vi "Admin.vi"(2 "Admin File Directory":string="C:\\Setup Files\\", 3 "MFC Error":u32) -> ()   [LabVIEW 2014]
uses:
  Program Files (x86)/National Instruments/LabVIEW 2014/examples/CompactRIO/Shared/cRIO Convert Thermocouple Readings.llb/Thermocouple Type.ctl
  <vilib>/Utility/file.llb/Read From Spreadsheet File (DBL).vi
  <vilib>/Utility/file.llb/Read From Spreadsheet File (string).vi
  <vilib>/Utility/file.llb/Write To Spreadsheet File (DBL).vi
  <vilib>/Utility/file.llb/Write To Spreadsheet File (string).vi
  <vilib>/Utility/file.llb/Write To Spreadsheet File (I64).vi
panel:
  in  "MKS 2":bool
  in  "IP Address MKS 2030 2":string
  in  "Mexa One":bool
  in  "IP Address Mexa One":string
  in  "Rapidox":bool
  in  "Mexa 584 - 2":bool
  in  "Mexa 584":bool
  out "PID Array":dbl[](array[numeric])
  out "Output array":u32[](array[numeric])
  out "IP array":string[](array[string])
  out "Boolean":bool
  in  "OK Button":bool
  in  "Tab Control":T1(tab)
  in  "Fast Warmup":bool
  in  "Omega":bool
  in  "Drive Cycle":bool
  in  "Ageing":bool
  in  "OSC Test":bool
  in  "AFR Sweep":bool
  in  "NO Light Off":bool
  in  "HC Light Off":bool
  in  "CO Light Off":bool
  in  "Heat Load Control":bool
  in  "Array Injection":bool
  in  "D SO2":dbl min=0.0 max=100.0
  in  "I SO2":dbl min=0.0 max=100.0
  in  "P SO2":dbl min=0.0 max=100.0
  in  "D NO":dbl min=0.0 max=100.0
  in  "I NO":dbl min=0.0 max=100.0
  in  "P NO":dbl min=0.0 max=100.0
  in  "D Fan":dbl min=0.0 max=100.0
  in  "I Fan":dbl min=0.0 max=100.0
  in  "P Fan":dbl min=0.0 max=100.0
  in  "D Furnace":dbl min=0.0 max=100.0
  in  "I Furnace":dbl min=0.0 max=100.0
  in  "P Furnace":dbl min=0.0 max=100.0
  in  "SO2 Loop":bool
  in  "CO2 Loop":bool
  in  "NO Loop":bool
  in  "Air Loop":bool
  in  "CO Loop":bool
  in  "HC Loop":bool
  in  "N2 Loop":bool
  in  "Air B Loop":bool
  in  "Air 2 Loop":bool
  in  "HC 2 Loop":bool
  in  "HC B Loop":bool
  out "CO -Al":bool
  out "HC - AL":bool
  out "AIR-Al":bool
  out "NO - AL":bool
  out "N2 - AL":bool
  out "SO2 AL":bool
  out "CO2 -Al":bool
  in  "HC-B Size":i32 min=0 max=100
  in  "Air-B Size":i32 min=0 max=5000
  in  "N2 Size":i32 min=0 max=1000
  in  "NO Size":i32 min=0 max=100
  in  "Air Size":i32 min=0 max=5000
  in  "HC Size":i32 min=0 max=100
  in  "CO Size":i32 min=0 max=100
  in  "N2-2 Size":i32 min=0 max=1000
  in  "Air-2 Size":i32 min=0 max=1000
  in  "HC-2 Size":i32 min=0 max=5000
  in  "O2 Size":i32 min=0 max=1000
  out "HC 2 - AL":bool
  out "Air 2 - AL":bool
  out "HC B -Al":bool
  out "Air B - AL":bool
  in  "SO2 F":bool
  in  "CO2 F":bool
  in  "NO F":bool
  in  "Air F":bool
  in  "CO F":bool
  in  "HC F":bool
  in  "N2 F":bool
  in  "Air B F":bool
  in  "Air 2 F":bool
  in  "HC 2 F":bool
  in  "HC B F":bool
  in  "HC-B":bool
  in  "N2":bool
  in  "NO":bool
  in  "Air":bool
  in  "CO":bool
  in  "HC":bool
  in  "Air-B":bool
  in  "Air-2":bool
  in  "HC-2":bool
  in  "O2":bool
  in  "N2-2":bool
  in  "Tank Thermocouple Limit":i32=300 min=0 max=1372
  in  "Heat Exch D":i32=1 min=0 max=32
  in  "Heat Exch C":i32=1 min=0 max=32
  in  "Heat Exch B":i32=1 min=0 max=32
  in  "Heat Exch A":i32=1 min=0 max=32
  in  "Vane Wheel":i32=1 min=0 max=32
  in  "Venturi":i32=1 min=0 max=32
  in  "Mopup Thermocouple":i32 min=0 max=32
  in  "Tank Thermocouple":i32 min=0 max=32
  in  "Process Thermocouple":i32=1 min=0 max=32
  in  "Process Thermocouple Limit":i32 min=0 max=1372
  in  "Bearing Temperature Limit":i32 min=0 max=200
  in  "Machine Temperature Limit":i32 min=0 max=1375
  in  "Bearing 1 TC":i32 min=0 max=32
  in  "Bearing 2 TC":i32 min=0 max=32
  in  "TC_Type_Array":T2[](array[typedef])=[3, 3, 3, 3, 3, 3, 3, 3, 3, 3, 3, 3, 3, 3, 3, 3] items=["B", "E", "J", "K", "R", "S", "T", "N"]
  in  "CO2 PS":bool
  in  "N2 PS":bool
  in  "CO PS":bool
  in  "HC PS":bool
  in  "Air-B/SO2 PS":bool
  in  "NO PS":bool
  in  "Air PS":bool
  in  "NO2 GLD":bool
  in  "SO2 GLD":bool
  in  "HC GLD":bool
  in  "CO GLD":bool
  in  "Inverter Err":bool
  in  "eStop":bool
  in  "ETAS":bool
  in  "IP Address ETAS":string
  in  "Port MKS":string
  in  "Port Mexa 7000-3":string
  in  "Port Mexa 7000-2":string
  in  "Port Mexa 7000-1":string
  in  "Mexa 7000-3":bool
  in  "IP Address Mexa 7000-3":string
  in  "Mexa 7000-2":bool
  in  "IP Address Mexa 7000-2":string
  in  "Mexa 7170":bool
  in  "MKS":bool
  in  "IP Address MKS 2030":string
  in  "IP Address Mexa 7000-1":string
  in  "Pressure Leak Test":i32 min=0 max=100
  in  "Delivery":i32 min=0 max=100
  in  "Air Bal":bool
  in  "N2 Leak":bool
  in  "Duration Leak Test":i32 min=0 max=100
  # "System Settings"
  # "Omicron"
  # "PID Settings"
  # "NO"
  # "Furnace"
  # "Fan"
  # "SO2"
  # "MFC Settings"
  # "Connected ?"
  # "Alarm"
  # "Size"
  # "Factors"
  # "Fast Loop"
  # "TC Settings"
  # "°C"
  # "°C"
  # "°C"
  # "°C"
  # "Flow Thermocouples"
  # "Heat Exchanger Thermocouples"
  # "TC Type"
  # "TC 01"
  # "TC 02"
  # "TC 03"
  # "When Selecting TC type PLEASE ensure the TC is wired with the correct wire back to the NI 9213 Module\n\nType: K Green (Default)\n          S Orange (Usually Furnace)\n          N Pink"
  # "TC 04"
  # "TC 05"
  # "TC 06"
  # "TC 07"
  # "TC 08"
  # "TC 09"
  # "TC 10"
  # "TC 11"
  # "TC 12"
  # "TC 13"
  # "TC 14"
  # "TC 15"
  # "TC 16"
  # "Alarm Settings"
  # "Analyser Settings"
  # "IP Address"
  # "Port Number"
  # "Leak Test Settings"
  # "KPa"
  # "s"
  # "l/min"
  # "Gas to be Used"
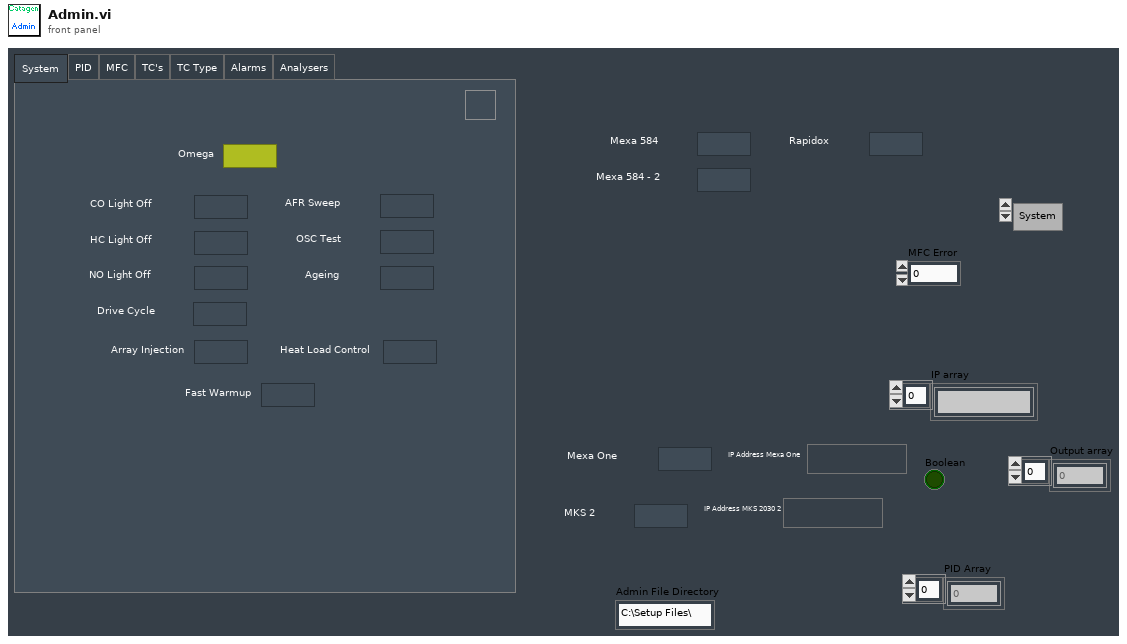
[diagram p1: front panel]
types:
  T1 = enum32{"System ", "Furnace", "MFC", "TC's", "TC Type", "Alarms", "Analysers", "Leak Test"}
  T2 = typedef "Thermocouple Type.ctl" = u16
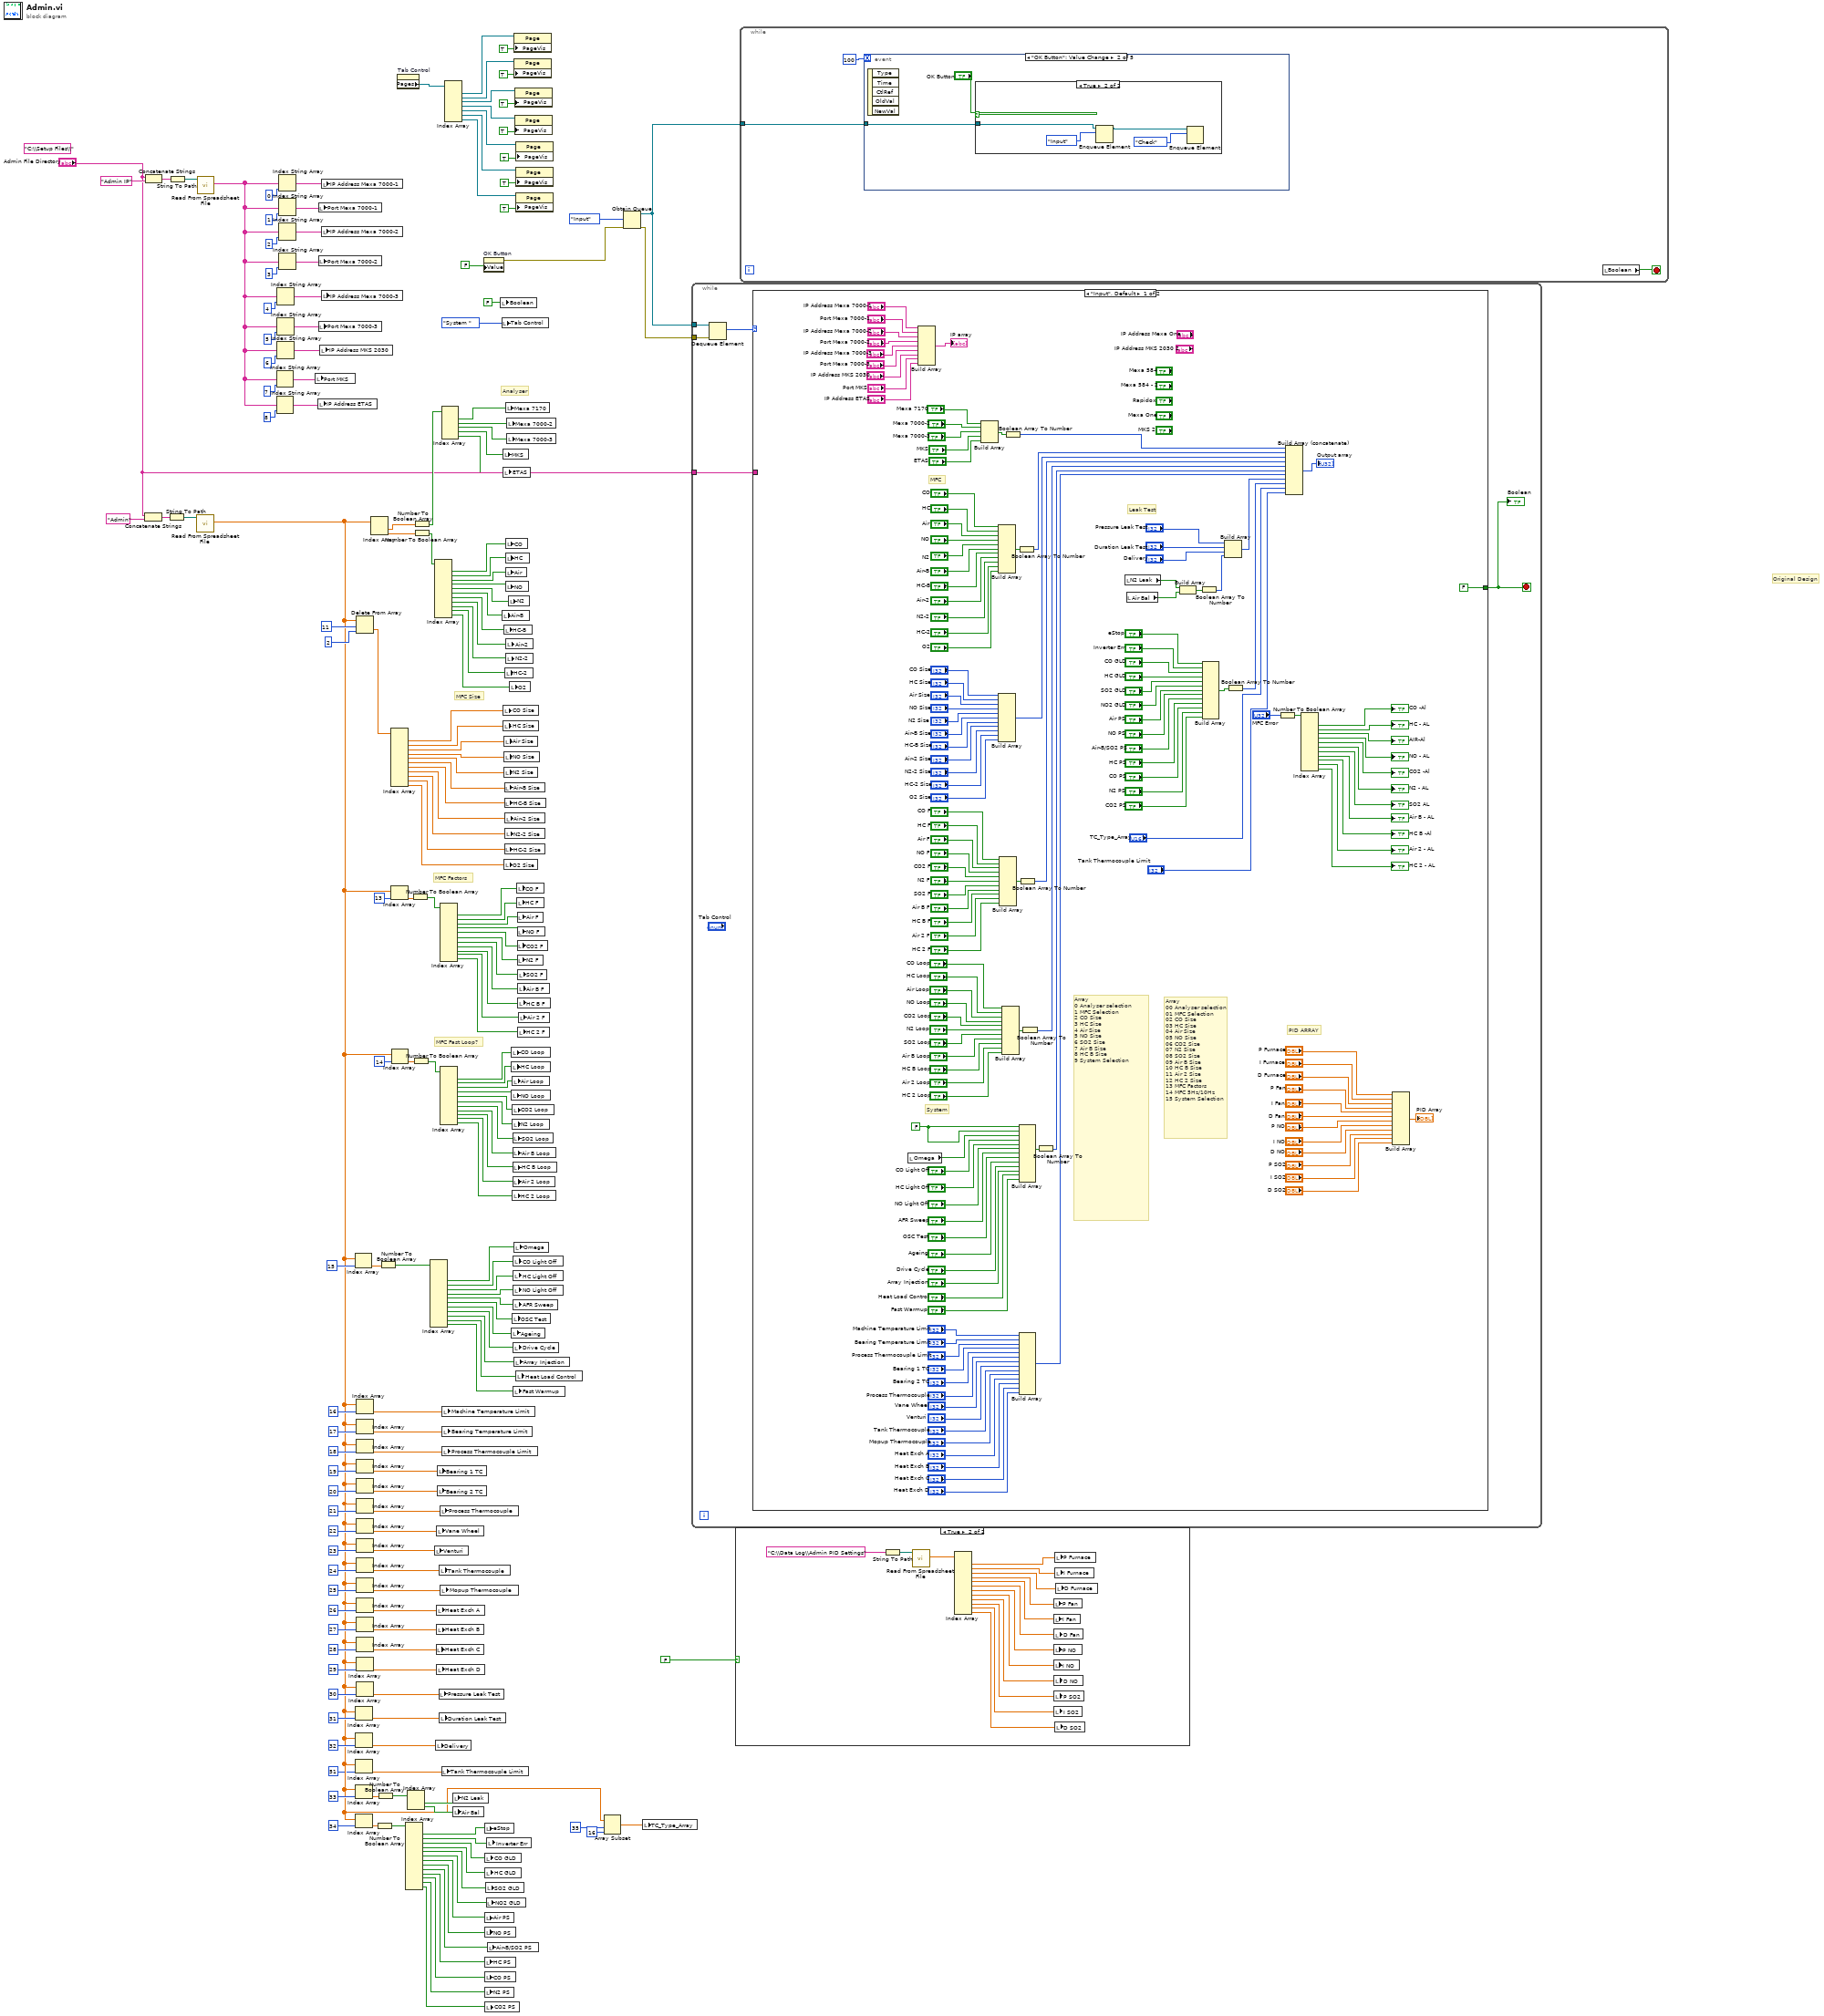
[diagram p0: block diagram]
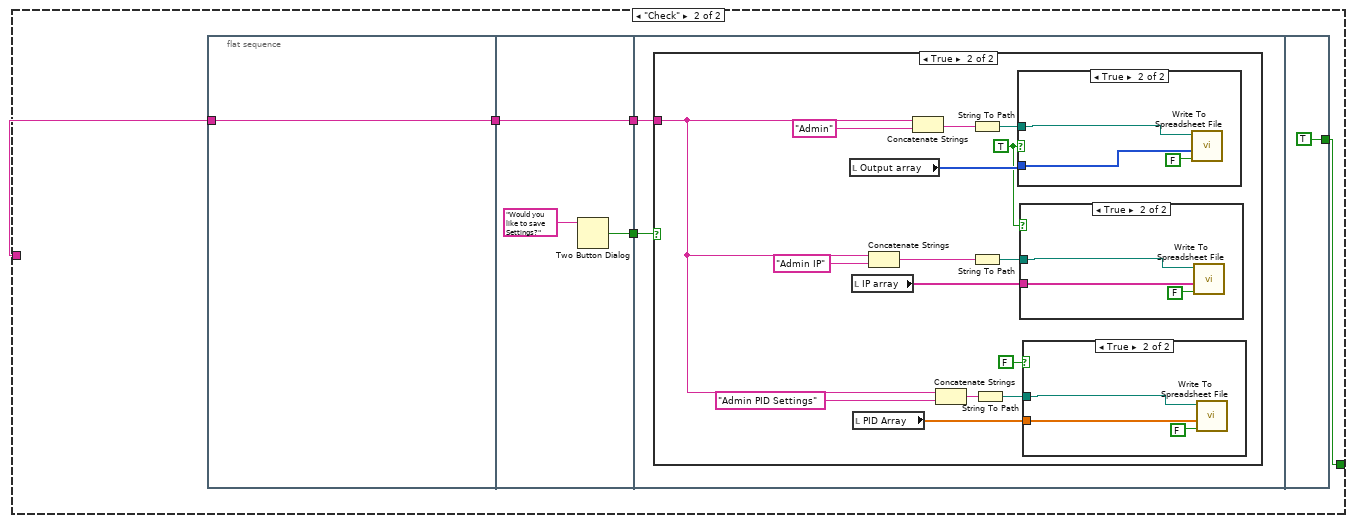
[diagram p3: hidden frame]
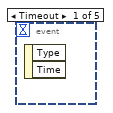
[diagram p8: hidden frame]
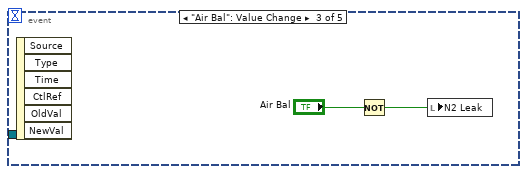
[diagram p10: hidden frame]
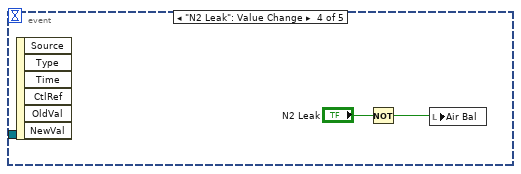
[diagram p11: hidden frame]
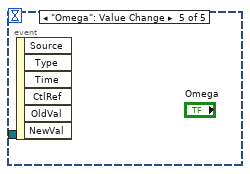
[diagram p12: hidden frame]
diagram:
  (unwired) "C:\\Setup Files\\" ("string")
  # "MFC Fast Loop?"
  # "MFC Factors"
  # "MFC Size"
  # "Analyser"
  # "Original Design"
  n1 = Concatenate Strings("Admin File Directory", "Admin" ("string")) -> (w50:string)
  n2 = Concatenate Strings("Admin File Directory", "Admin IP" ("string")) -> (w53:string)
  n3 = String To Path(string=w50) -> (path=w49:path)
  n4 = String To Path(string=w53) -> (path=w155:path)
  n5 = call-poly <vilib>:"Read From Spreadsheet File.vi"("file path (dialog if empty)"=w49) -> ("first row"=w2:dbl[])  [unwired: 6 in, 4 out]
  n6 = call-poly <vilib>:"Read From Spreadsheet File.vi"("file path (dialog if empty)"=w155) -> ("first row"=w9:string[])  [unwired: 6 in, 4 out]
  n7 = Index String Array(1:7 ("index"), 2:w9) -> (0:w10:string)  [unwired: 1 in]
  n8 = Index String Array(1:8 ("index"), 2:w9) -> (0:w8:string)  [unwired: 1 in]
  n9 = Index String Array(1:4 ("index"), 2:w9) -> (0:w65:string)  [unwired: 1 in]
  n10 = Index String Array(1:5 ("index"), 2:w9) -> (0:w67:string)  [unwired: 1 in]
  n11 = Index String Array(1:6 ("index"), 2:w9) -> (0:w63:string)  [unwired: 1 in]
  n12 = Index String Array(1:0 ("index"), 2:w9) -> (0:w150:string)  [unwired: 1 in]
  n13 = Index String Array(1:1 ("index"), 2:w9) -> (0:w151:string)  [unwired: 1 in]
  n14 = Index String Array(1:2 ("index"), 2:w9) -> (0:w124:string)  [unwired: 1 in]
  n15 = Index String Array(1:3 ("index"), 2:w9) -> (0:w126:string)  [unwired: 1 in]
  n16 = local write "Port MKS"(w10) -> ()
  n17 = local write "IP Address ETAS"(w8) -> ()
  n18 = local write "Port Mexa 7000-1"(w151) -> ()
  n19 = local write "Port Mexa 7000-2"(w126) -> ()
  n20 = local write "Port Mexa 7000-3"(w67) -> ()
  n21 = local write "IP Address MKS 2030"(w63) -> ()
  n22 = local write "IP Address Mexa 7000-1"(w150) -> ()
  n23 = local write "IP Address Mexa 7000-2"(w124) -> ()
  n24 = local write "IP Address Mexa 7000-3"(w65) -> ()
  n25 = Index Array(array=w2, index=15) -> (element=w121:dbl)
  n26 = Index Array(array=w2, index=31) -> (element=w85:dbl)
  n27 = Index Array(array=w2, index=32) -> (element=w84:dbl)
  n28 = Index Array(array=w2, index=51) -> (element=w3:dbl)
  n29 = Index Array(array=w2, index=33) -> (element=w91:dbl)
  n30 = Index Array(array=w2, index=34) -> (element=w27:dbl)
  n31 = Index Array(array=w2, index=30) -> (element=w86:dbl)
  n32 = Delete From Array(array=w2, length=11, index=2) -> (deleted portion=w180:dbl[])  [unwired: 1 out]
  n33 = Index Array(array=w2, index=16) -> (element=w88:dbl)
  n34 = Index Array(array=w2, index=17) -> (element=w87:dbl)
  n35 = Index Array(array=w2, index=18) -> (element=w60:dbl)
  n36 = Index Array(array=w2, index=19) -> (element=w61:dbl)
  n37 = Index Array(array=w2, index=20) -> (element=w54:dbl)
  n38 = Index Array(array=w2, index=21) -> (element=w55:dbl)
  n39 = Index Array(array=w2, index=22) -> (element=w38:dbl)
  n40 = Index Array(array=w2, index=23) -> (element=w40:dbl)
  n41 = Index Array(array=w2, index=24) -> (element=w39:dbl)
  n42 = Index Array(array=w2, index=25) -> (element=w46:dbl)
  n43 = Index Array(array=w2, index=26) -> (element=w45:dbl)
  n44 = Index Array(array=w2, index=27) -> (element=w31:dbl)
  n45 = Index Array(array=w2, index=28) -> (element=w32:dbl)
  n46 = Index Array(array=w2, index=29) -> (element=w33:dbl)
  n47 = Index Array(array=w2) -> (element #1=w184:dbl, element #2=w182:dbl)  [unwired: 2 in]
  n48 = Number To Boolean Array(number=w27) -> (Boolean array=w26:bool[])
  n49 = Number To Boolean Array(number=w91) -> (Boolean array=w89:bool[])
  n50 = Number To Boolean Array(number=w121) -> (Boolean array=w123:bool[])
  n51 = Index Array(array=w180) -> (element #1=w166:dbl, element #2=w165:dbl, element #3=w164:dbl, element #4=w163:dbl, element #5=w162:dbl, element #6=w161:dbl, element #7=w160:dbl, element #8=w144:dbl, element #9=w143:dbl, element #10=w142:dbl, element #11=w141:dbl)  [unwired: 11 in]
  n52 = Index Array(array=w2, index=13) -> (element=w140:dbl)
  n53 = Index Array(array=w2, index=14) -> (element=w107:dbl)
  n54 = property on="Tab Control" class="TabCtl (strict)"() -> ("Pages"=w81:refnum<vi>[])  [unwired: 2 in, 2 out]
  n55 = Index Array(array=w26) -> (element #1=w25:bool, element #2=w24:bool, element #3=w23:bool, element #4=w22:bool, element #5=w21:bool, element #6=w20:bool, element #7=w19:bool, element #8=w18:bool, element #9=w17:bool, element #10=w16:bool, element #11=w15:bool, element #12=w14:bool, element #13=w13:bool)  [unwired: 13 in]
  n56 = Index Array(array=w89) -> (element #1=w83:bool, element #2=w82:bool)  [unwired: 2 in]
  n57 = Number To Boolean Array(number=w140) -> (Boolean array=w138:bool[])
  n58 = Number To Boolean Array(number=w107) -> (Boolean array=w109:bool[])
  n59 = Number To Boolean Array(number=w184) -> (Boolean array=w183:bool[])
  n60 = Number To Boolean Array(number=w182) -> (Boolean array=w181:bool[])
  n61 = Index Array(array=w123) -> (element #3=w106:bool, element #4=w105:bool, element #5=w104:bool, element #6=w103:bool, element #7=w102:bool, element #8=w101:bool, element #9=w100:bool, element #10=w99:bool, element #11=w98:bool, element #12=w97:bool, element #13=w47:bool)  [unwired: 13 in, 2 out]
  n62 = local write "Venturi"(w40) -> ()
  n63 = Index Array(array=w181) -> (element #1=w177:bool, element #2=w176:bool, element #3=w175:bool, element #4=w174:bool, element #5=w173:bool, element #6=w172:bool, element #7=w171:bool, element #8=w148:bool, element #9=w147:bool, element #10=w146:bool, element #11=w145:bool)  [unwired: 11 in]
  n64 = local write "Delivery"(w84) -> ()
  n65 = local write "Heat Exch C"(w32) -> ()
  n66 = local write "Vane Wheel"(w38) -> ()
  n67 = local write "Heat Exch A"(w45) -> ()
  n68 = local write "Heat Exch B"(w31) -> ()
  n69 = local write "Heat Exch D"(w33) -> ()
  n70 = local write "Bearing 1 TC"(w61) -> ()
  n71 = local write "Bearing 2 TC"(w54) -> ()
  n72 = local write "Pressure Leak Test"(w86) -> ()
  n73 = local write "Tank Thermocouple"(w39) -> ()
  n74 = local write "Duration Leak Test"(w85) -> ()
  n75 = Index Array(array=w138) -> (element #1=w137:bool, element #2=w136:bool, element #3=w135:bool, element #4=w134:bool, element #5=w133:bool, element #6=w132:bool, element #7=w131:bool, element #8=w130:bool, element #9=w129:bool, element #10=w128:bool, element #11=w127:bool)  [unwired: 11 in]
  n76 = local write "Process Thermocouple"(w55) -> ()
  n77 = Index Array(array=w109) -> (element #1=w110:bool, element #2=w111:bool, element #3=w112:bool, element #4=w113:bool, element #5=w114:bool, element #6=w115:bool, element #7=w116:bool, element #8=w117:bool, element #9=w118:bool, element #10=w119:bool, element #11=w120:bool)  [unwired: 11 in]
  n78 = local write "Mopup Thermocouple"(w46) -> ()
  n79 = Index Array(array=w183) -> (element #1=w170:bool, element #2=w169:bool, element #3=w168:bool, element #4=w167:bool, element #5=w12:bool)  [unwired: 5 in]
  n80 = local write "Tank Thermocouple Limit"(w3) -> ()
  n81 = local write "Machine Temperature Limit"(w88) -> ()
  n82 = local write "Bearing Temperature Limit"(w87) -> ()
  n83 = local write "Process Thermocouple Limit"(w60) -> ()
  n84 = Index Array(array=w81) -> (element #1=w80:refnum<vi>, element #2=w79:refnum<vi>, element #3=w78:refnum<vi>, element #4=w77:refnum<vi>, element #5=w76:refnum<vi>, element #6=w75:refnum<vi>, element #7=w29:refnum<vi>)  [unwired: 7 in]
  n85 = local write "N2 Leak"(w83) -> ()
  n86 = local write "Air Bal"(w82) -> ()
  n87 = property on="OK Button" class="Bool (strict)"("Value"=FALSE ("OK Button")) -> (error out=w158:errorcluster)  [unwired: 2 in, 1 out]
  n88 = local write "eStop"(w25) -> ()
  n89 = local write "Air PS"(w19) -> ()
  n90 = local write "NO PS"(w18) -> ()
  n91 = local write "HC PS"(w16) -> ()
  n92 = local write "CO PS"(w15) -> ()
  n93 = local write "N2 PS"(w14) -> ()
  n94 = local write "CO GLD"(w23) -> ()
  n95 = local write "HC GLD"(w22) -> ()
  n96 = local write "CO2 PS"(w13) -> ()
  n97 = local write "SO2 GLD"(w21) -> ()
  n98 = local write "NO2 GLD"(w20) -> ()
  n99 = local write "Inverter Err"(w24) -> ()
  n100 = local write "Air-B/SO2 PS"(w17) -> ()
  n101 = local write "Boolean"(FALSE ("Boolean")) -> ()
  n102 = local write "Tab Control"(T1."System " ("Tab Control")) -> ()
  n103 = local write "Air-B"(w172) -> ()
  n104 = local write "MKS"(w167) -> ()
  n105 = local write "ETAS"(w12) -> ()
  n106 = local write "CO Size"(w166) -> ()
  n107 = local write "HC Size"(w165) -> ()
  n108 = local write "HC-B"(w171) -> ()
  n109 = local write "Air Size"(w164) -> ()
  n110 = local write "NO Size"(w163) -> ()
  n111 = local write "N2 Size"(w162) -> ()
  n112 = local write "O2 Size"(w141) -> ()
  n113 = local write "Air-B Size"(w161) -> ()
  n114 = local write "HC-B Size"(w160) -> ()
  n115 = local write "HC-2 Size"(w142) -> ()
  n116 = local write "HC-2"(w146) -> ()
  n117 = local write "Air-2 Size"(w144) -> ()
  n118 = local write "N2-2 Size"(w143) -> ()
  n119 = local write "Mexa 7170"(w170) -> ()
  n120 = local write "CO"(w177) -> ()
  n121 = local write "HC"(w176) -> ()
  n122 = local write "Air"(w175) -> ()
  n123 = local write "NO"(w174) -> ()
  n124 = local write "Air-2"(w148) -> ()
  n125 = local write "N2-2"(w147) -> ()
  n126 = local write "Mexa 7000-2"(w169) -> ()
  n127 = local write "Mexa 7000-3"(w168) -> ()
  n128 = local write "N2"(w173) -> ()
  n129 = local write "O2"(w145) -> ()
  n130 = local write "CO Loop"(w110) -> ()
  n131 = local write "HC Loop"(w111) -> ()
  n132 = local write "NO Loop"(w113) -> ()
  n133 = local write "Ageing"(w100) -> ()
  n134 = local write "Air Loop"(w112) -> ()
  n135 = local write "CO2 Loop"(w114) -> ()
  n136 = local write "N2 Loop"(w115) -> ()
  n137 = local write "HC 2 Loop"(w120) -> ()
  n138 = local write "OSC Test"(w101) -> ()
  n139 = local write "SO2 Loop"(w116) -> ()
  n140 = local write "Air B Loop"(w117) -> ()
  n141 = local write "HC B Loop"(w118) -> ()
  n142 = local write "Air 2 Loop"(w119) -> ()
  n143 = local write "CO Light Off"(w105) -> ()
  n144 = local write "HC Light Off"(w104) -> ()
  n145 = local write "NO Light Off"(w103) -> ()
  n146 = local write "AFR Sweep"(w102) -> ()
  n147 = local write "Drive Cycle"(w99) -> ()
  n148 = local write "Fast Warmup"(w47) -> ()
  n149 = property class="Page"(reference=w80, "PageVis"=TRUE ("Page Visible")) -> ()  [unwired: 1 in, 2 out]
  n150 = property class="Page"(reference=w79, "PageVis"=TRUE ("Page Visible")) -> ()  [unwired: 1 in, 2 out]
  n151 = local write "Omega"(w106) -> ()
  n152 = local write "Array Injection"(w98) -> ()
  n153 = property class="Page"(reference=w78, "PageVis"=TRUE ("Page Visible")) -> ()  [unwired: 1 in, 2 out]
  n154 = property class="Page"(reference=w77, "PageVis"=TRUE ("Page Visible")) -> ()  [unwired: 1 in, 2 out]
  n155 = property class="Page"(reference=w76, "PageVis"=TRUE ("Page Visible")) -> ()  [unwired: 1 in, 2 out]
  n156 = property class="Page"(reference=w75, "PageVis"=TRUE ("Page Visible")) -> ()  [unwired: 1 in, 2 out]
  n157 = property class="Page"(reference=w29, "PageVis"=TRUE ("Page Visible")) -> ()  [unwired: 1 in, 2 out]
  n158 = local write "Heat Load Control"(w97) -> ()
  n159 = local write "CO F"(w137) -> ()
  n160 = local write "HC F"(w136) -> ()
  n161 = local write "Air F"(w135) -> ()
  n162 = local write "NO F"(w134) -> ()
  n163 = local write "CO2 F"(w133) -> ()
  n164 = local write "N2 F"(w132) -> ()
  n165 = local write "SO2 F"(w131) -> ()
  n166 = local write "Air B F"(w130) -> ()
  n167 = local write "HC B F"(w129) -> ()
  n168 = local write "HC 2 F"(w127) -> ()
  n169 = local write "Air 2 F"(w128) -> ()
  n170 = Array Subset(array=w2, index=35, length=16) -> (w4:dbl[])
  n171 = Obtain Queue(element data type=enum16{"Input", "Check"}."Input", error in (no error)=w158) -> (queue out=w185:refnum<queue>, error out=w157:errorcluster)  [unwired: 3 in, 1 out]
  n172 = local write "TC_Type_Array"(w4) -> ()
  n173 = while {
    tunnel: w185 -> [w191]
    tunnel: w157 -> [w188]
    tunnel: "Admin File Directory" -> [w187]
    stop <- w189 stop-if-true
    n174 = Dequeue Element(queue=w191, error in (no error)=w188) -> (element=w190:enum16{"Input", "Check"})  [unwired: 1 in, 3 out]
    n175 = case shown="\"Input\", Default" w190 {
      tunnel: [FALSE w346] -> w189
      tunnel: w187 -> [_ w344]
      frame "Input", Default {
        w193 = FALSE ("element")
        # "Array\n00 Analyser selection\n01 MFC Selection\n02 CO Size\n03 HC Size\n04 Air Size\n05 NO Size\n06 CO2 Size\n07 N2 Size\n08 SO2 Size\n09 Air B Size\n10 HC B Size\n11 Air 2 Size\n12 HC 2 Size\n13 MFC Factors\n14 MFC 5Hz/10Hz\n15 System Selection"
        # "Array\n0 Analyser selection\n1 MFC Selection\n2 CO Size\n3 HC Size\n4 Air Size\n5 NO Size\n6 SO2 Size\n7 Air B Size\n8 HC B Size\n9 System Selection"
        # "PID ARRAY"
        # "System"
        # "MFC"
        # "Leak Test"
        n176 = local read "Omega"() -> (w241:bool)
        n177 = Build Array("IP Address Mexa 7000-1", "Port Mexa 7000-1", "IP Address Mexa 7000-2", "Port Mexa 7000-2", "IP Address Mexa 7000-3", "Port Mexa 7000-3", "IP Address MKS 2030", "Port MKS", "IP Address ETAS") -> (→"IP array":string[])
        n178 = Build Array("Mexa 7170", "Mexa 7000-2", "Mexa 7000-3", "MKS", "ETAS") -> (w340:bool[])
        n179 = Build Array("CO", "HC", "Air", "NO", "N2", "Air-B", "HC-B", "Air-2", "N2-2", "HC-2", "O2") -> (w332:bool[])
        n180 = Build Array("CO Size", "HC Size", "Air Size", "NO Size", "N2 Size", "Air-B Size", "HC-B Size", "Air-2 Size", "N2-2 Size", "HC-2 Size", "O2 Size") -> (w322:i32[])
        n181 = Build Array("CO F", "HC F", "Air F", "NO F", "CO2 F", "N2 F", "SO2 F", "Air B F", "HC B F", "Air 2 F", "HC 2 F") -> (w288:bool[])
        n182 = Build Array("CO Loop", "HC Loop", "Air Loop", "NO Loop", "CO2 Loop", "N2 Loop", "SO2 Loop", "Air B Loop", "HC B Loop", "Air 2 Loop", "HC 2 Loop") -> (w264:bool[])
        n183 = Boolean Array To Number(Boolean array=w340) -> (number=w324:u32)
        n184 = Boolean Array To Number(Boolean array=w332) -> (number=w323:u32)
        n185 = Build Array(w193, w193, w241, "CO Light Off", "HC Light Off", "NO Light Off", "AFR Sweep", "OSC Test", "Ageing", "Drive Cycle", "Array Injection", "Heat Load Control", "Fast Warmup") -> (w310:bool[])
        n186 = Build Array("Machine Temperature Limit", "Bearing Temperature Limit", "Process Thermocouple Limit", "Bearing 1 TC", "Bearing 2 TC", "Process Thermocouple", "Vane Wheel", "Venturi", "Tank Thermocouple", "Mopup Thermocouple", "Heat Exch A", "Heat Exch B", "Heat Exch C", "Heat Exch D") -> (w242:i32[])
        n187 = Boolean Array To Number(Boolean array=w288) -> (number=w276:u32)
        n188 = Boolean Array To Number(Boolean array=w264) -> (number=w252:u32)
        n189 = Boolean Array To Number(Boolean array=w310) -> (number=w275:u32)
        n190 = local read "N2 Leak"() -> (w270:bool)
        n191 = local read "Air Bal"() -> (w269:bool)
        n192 = Build Array(w270, w269) -> (w268:bool[])
        n193 = Boolean Array To Number(Boolean array=w268) -> (number=w266:u32)
        n194 = Build Array("eStop", "Inverter Err", "CO GLD", "HC GLD", "SO2 GLD", "NO2 GLD", "Air PS", "NO PS", "Air-B/SO2 PS", "HC PS", "CO PS", "N2 PS", "CO2 PS") -> (w211:bool[])
        n195 = Build Array("Pressure Leak Test", "Duration Leak Test", "Delivery", w266) -> (w237:u32[])
        n196 = Boolean Array To Number(Boolean array=w211) -> (number=w210:u32)
        n197 = Number To Boolean Array(number="MFC Error") -> (Boolean array=w316:bool[])
        n198 = Build Array (concatenate)(w324, w323, w322, w276, w252, w275, w242, w237, w210, "TC_Type_Array", "Tank Thermocouple Limit") -> (→"Output array":u32[])
        n199 = Index Array(array=w316) -> (element #1=→"CO -Al":bool, element #2=→"HC - AL":bool, element #3=→"AIR-Al":bool, element #4=→"NO - AL":bool, element #5=→"CO2 -Al":bool, element #6=→"N2 - AL":bool, element #7=→"SO2 AL":bool, element #8=→"Air B - AL":bool, element #9=→"HC B -Al":bool, element #10=→"Air 2 - AL":bool, element #11=→"HC 2 - AL":bool)  [unwired: 11 in]
        n200 = Build Array("P Furnace", "I Furnace", "D Furnace", "P Fan", "I Fan", "D Fan", "P NO", "I NO", "D NO", "P SO2", "I SO2", "D SO2") -> (→"PID Array":dbl[])
      }
      frame "Check" {
        n201 = flat-sequence {
          tunnel: w344 -> [w347]
          tunnel: [w347] -> w343
          tunnel: [w349] -> w345
          tunnel: w343 -> [w348]
          tunnel: [w348] -> w342
          tunnel: w345 -> [w352]
          tunnel: w342 -> [w351]
          tunnel: [TRUE] -> w346
          frame #0 {
          }
          frame #1 {
            n202 = Two Button Dialog(message="Would you like to save Settings?") -> (T button?=w349:bool)  [unwired: 2 in]
          }
          frame #2 {
            n203 = case shown="True" w352 {
              tunnel: w351 -> [_ w353]
              frame False {
              }
              frame True {
                w361 = TRUE
                n204 = local read "Output array"() -> (w366:u32[])
                n205 = local read "IP array"() -> (w364:string[])
                n206 = local read "PID Array"() -> (w363:dbl[])
                n207 = Concatenate Strings(w353, "Admin IP" ("string")) -> (w357:string)
                n208 = Concatenate Strings(w353, "Admin" ("string")) -> (w355:string)
                n209 = Concatenate Strings(w353, "Admin PID Settings" ("string")) -> (w359:string)
                n210 = String To Path(string=w355) -> (path=w367:path)
                n211 = String To Path(string=w357) -> (path=w365:path)
                n212 = String To Path(string=w359) -> (path=w362:path)
                n213 = case shown="True" w361 {
                  tunnel: w366 -> [_ w375]
                  tunnel: w367 -> [_ w374]
                  frame False {
                  }
                  frame True {
                    n214 = call-poly <vilib>:"Write To Spreadsheet File.vi"("append to file? (new file:F)"=FALSE, "1D data"=w375, "file path (dialog if empty)"=w374) -> ()  [unwired: 5 in, 1 out]
                  }
                }
                n215 = case shown="True" w361 {
                  tunnel: w365 -> [_ w372]
                  tunnel: w364 -> [_ w371]
                  frame False {
                  }
                  frame True {
                    n216 = call-poly <vilib>:"Write To Spreadsheet File.vi"("append to file? (new file:F)"=FALSE, "1D data"=w371, "file path (dialog if empty)"=w372) -> ()  [unwired: 5 in, 1 out]
                  }
                }
                n217 = case shown="True" FALSE {
                  tunnel: w362 -> [_ w369]
                  tunnel: w363 -> [_ w368]
                  frame False {
                  }
                  frame True {
                    n218 = call-poly <vilib>:"Write To Spreadsheet File.vi"("append to file? (new file:F)"=FALSE, "1D data"=w368, "file path (dialog if empty)"=w369) -> ()  [unwired: 5 in, 1 out]
                  }
                }
              }
            }
          }
          frame #3 {
          }
        }
      }
    }
    "Boolean" <- w189
  }
  n219 = case shown="True" FALSE {
    frame False {
    }
    frame True {
      n220 = String To Path(string="C:\\Data Log\\Admin PID Settings") -> (path=w392:path)
      n221 = call-poly <vilib>:"Read From Spreadsheet File.vi"("file path (dialog if empty)"=w392) -> ("first row"=w390:dbl[])  [unwired: 6 in, 4 out]
      n222 = Index Array(array=w390) -> (element #1=w389:dbl, element #2=w388:dbl, element #3=w387:dbl, element #4=w386:dbl, element #5=w385:dbl, element #6=w384:dbl, element #7=w383:dbl, element #8=w382:dbl, element #9=w381:dbl, element #10=w380:dbl, element #11=w379:dbl, element #12=w378:dbl)  [unwired: 12 in]
      n223 = local write "P Fan"(w386) -> ()
      n224 = local write "I Fan"(w385) -> ()
      n225 = local write "P NO"(w383) -> ()
      n226 = local write "I NO"(w382) -> ()
      n227 = local write "D Fan"(w384) -> ()
      n228 = local write "D NO"(w381) -> ()
      n229 = local write "P SO2"(w380) -> ()
      n230 = local write "I SO2"(w379) -> ()
      n231 = local write "P Furnace"(w389) -> ()
      n232 = local write "I Furnace"(w388) -> ()
      n233 = local write "D SO2"(w378) -> ()
      n234 = local write "D Furnace"(w387) -> ()
    }
  }
  n235 = while {
    tunnel: w185 -> [w394]
    stop <- w393 stop-if-true
    n236 = event shown="[1] \"OK Button\": Value Change" {
      selector: _ -> [_ _ _ _ _]
      dyn-events: _ -> [_ _ _ _ _]
      timeout: 100 -> [_ _ _ _ _]
      tunnel: w394 -> [_ w397 _ _ _]
      event Timeout {
        n237 = event-data() -> ()  [unwired: 1 in, 2 out]
      }
      event "OK Button": Value Change {
        n238 = event-data() -> ()  [unwired: 1 in, 5 out]
        n239 = case shown="True" "OK Button" {
          tunnel: w397 -> [_ w399]
          frame False {
          }
          frame True {
            n240 = Enqueue Element(queue=w399, element=enum16{"Input", "Check"}."Input") -> (queue out=w398:refnum<queue>)  [unwired: 2 in, 2 out]
            n241 = Enqueue Element(queue=w398, element=enum16{"Input", "Check"}."Check") -> ()  [unwired: 2 in, 3 out]
          }
        }
      }
      event "Air Bal": Value Change {
        n242 = event-data() -> ()  [unwired: 1 in, 6 out]
        n243 = Not(x="Air Bal") -> (.not. x?=w403:bool)
        n244 = local write "N2 Leak"(w403) -> ()
      }
      event "N2 Leak": Value Change {
        n245 = event-data() -> ()  [unwired: 1 in, 6 out]
        n246 = Not(x="N2 Leak") -> (.not. x?=w404:bool)
        n247 = local write "Air Bal"(w404) -> ()
      }
      event "Omega": Value Change {
        n248 = event-data() -> ()  [unwired: 1 in, 6 out]
      }
    }
    n249 = local read "Boolean"() -> (w393:bool)
  }
